vi "PS CONTROL TEST.vi"() -> ()   [LabVIEW 2019]
panel:
  in  "stop":bool
  in  "Power Supply State":T1(ring)
  out "Field [T]":dbl format="%.4f"
  in  "Ramp to Zero":bool
  in  "Hold":bool
  in  "Ramp to Setpoint":bool
  in  "Rate [T/min]":dbl min=0.0 max=5.0 step=0.1 format="%.5f"
  in  "Setpoint [T]":dbl format="%.5f"
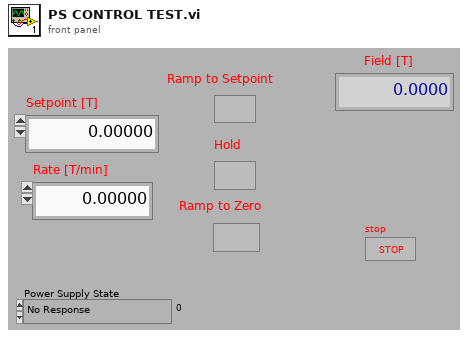
[diagram p1: front panel]
types:
  T1 = enum16{"No Response", "Ramping to programmed field ", "Holding at programmed field", "Paused", "Ramp Manual Up", "Ramp Manual Down", "Ramping to Zero", "QUENCH", "Heating Persistance Switch", "At Zero Current"}
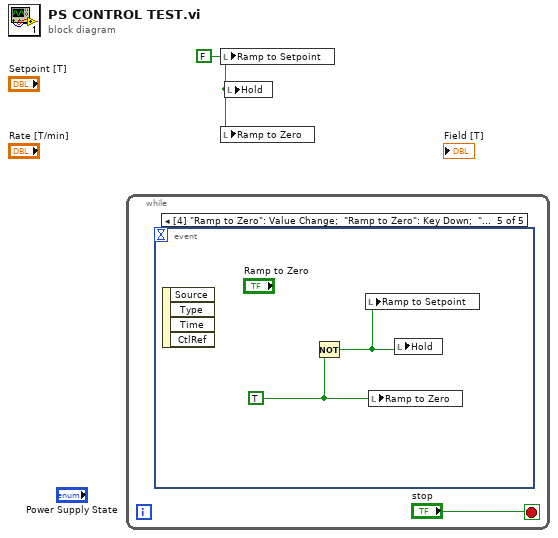
[diagram p0: block diagram]
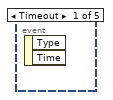
[diagram p2: hidden frame]
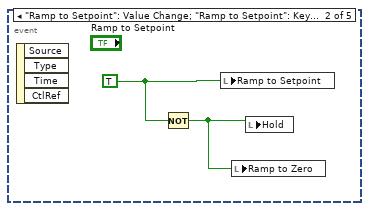
[diagram p3: hidden frame]
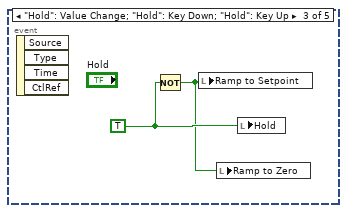
[diagram p4: hidden frame]
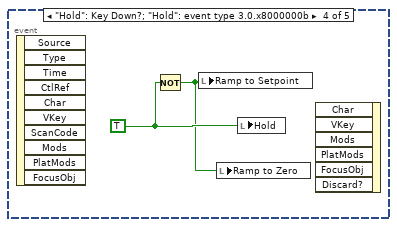
[diagram p5: hidden frame]
diagram:
  w1 = FALSE ("Ramp to Setpoint")
  n1 = while {
    stop <- "stop" stop-if-true
    n2 = event shown="[4] \"Ramp to Zero\": Value Change;  \"Ramp to Zero\": Key Down;  \"Ramp to Zero\": Key Up" {
      selector: _ -> [_ _ _ _ _]
      dyn-events: _ -> [_ _ _ _ _]
      timeout: _ -> [_ _ _ _ _]
      event Timeout {
        n3 = event-data() -> ()  [unwired: 1 in, 2 out]
      }
      event "Ramp to Setpoint": Value Change; "Ramp to Setpoint": Key Down; "Ramp to Setpoint": Key Up {
        w3 = TRUE ("Ramp to Setpoint")
        n4 = event-data() -> ()  [unwired: 1 in, 4 out]
        n5 = Not(x=w3) -> (.not. x?=w4:bool)
        n6 = local write "Ramp to Setpoint"(w3) -> ()
        n7 = local write "Ramp to Zero"(w4) -> ()
        n8 = local write "Hold"(w4) -> ()
      }
      event "Hold": Value Change; "Hold": Key Down; "Hold": Key Up {
        w6 = TRUE ("Hold")
        n9 = event-data() -> ()  [unwired: 1 in, 4 out]
        n10 = Not(x=w6) -> (.not. x?=w5:bool)
        n11 = local write "Ramp to Setpoint"(w5) -> ()
        n12 = local write "Ramp to Zero"(w5) -> ()
        n13 = local write "Hold"(w6) -> ()
      }
      event "Hold": Key Down?; "Hold": event type 3.0.x8000000b {
        w8 = TRUE ("Hold")
        n14 = event-data() -> ()  [unwired: 1 in, 10 out]
        n15 = Not(x=w8) -> (.not. x?=w7:bool)
        n16 = local write "Ramp to Setpoint"(w7) -> ()
        n17 = local write "Ramp to Zero"(w7) -> ()
        n18 = local write "Hold"(w8) -> ()
        n19 = event-data() -> ()  [unwired: 7 in, 1 out]
      }
      event "Ramp to Zero": Value Change; "Ramp to Zero": Key Down; "Ramp to Zero": Key Up {
        w10 = TRUE ("Ramp to Zero")
        n20 = event-data() -> ()  [unwired: 1 in, 4 out]
        n21 = Not(x=w10) -> (.not. x?=w9:bool)
        n22 = local write "Ramp to Setpoint"(w9) -> ()
        n23 = local write "Ramp to Zero"(w10) -> ()
        n24 = local write "Hold"(w9) -> ()
      }
    }
  }
  n25 = local write "Ramp to Setpoint"(w1) -> ()
  n26 = local write "Ramp to Zero"(w1) -> ()
  n27 = local write "Hold"(w1) -> ()
